vi "Actor Core.vi"(8 "error in":errorcluster, 11 "Activation in":refnum<class "Activation.lvclass">) -> (0 "error out":errorcluster, 3 "Actor out":refnum<class "Actor.lvclass">)   [LabVIEW 2018, in "Activation Actor.lvlib" / "Activation.lvclass"]
doc: "(<B>Filename</B>: Actor Framework.lvlib:Actor.lvclass:Actor Core.vi)\n\nReceives messages to the actor, reacts to them, and initiates any error handling that may shut the actor down.\n\nDescendant classes may override this VI to append parallel tasks for the actor to complete while it handles messages. Overrides use the Call Parent Method node."
uses:
  Activation.lvclass
  C:/Users/Administrator/Desktop/LabVIEW EMS/EMS Generic Actor/EMS Generic/EMS Generic.lvclass
  C:/Users/Administrator/Desktop/LabVIEW EMS/Device Communication and Control Abstract Actor/Device Communication and Control Abstract/Device Communication and Control Abstract.lvclass
  C:/Users/Administrator/Desktop/LabVIEW EMS/Optimization/Startup Optimization Actor/Startup Optimization/Startup Optimization.lvclass
  C:/Users/Administrator/Desktop/LabVIEW EMS/Optimization/Generic Optimization Actor/Generic Optimization/Generic Optimization.lvclass
  C:/Program Files (x86)/National Instruments/LabVIEW 2018/vi.lib/ActorFramework/Actor/Actor.lvclass
  <vilib>/ActorFramework/Actor/Actor.lvclass
  Controls/Activation State.ctl
  <vilib>/ORNL/CSEISMIC DDS/CSEISMIC DDS Base/Data Types/Controls/DeviceID.ctl
  EMS Generic Actor/EMS Generic/EMS Generic.lvclass/EMS Generic.ctl
  EMS Generic Actor/EMS Generic/Controls/Device Information Cluster.ctl
  EMS Generic Actor/EMS Generic/Controls/Device State.ctl
  <vilib>/ORNL/CSEISMIC DDS/CSEISMIC DDS Base/Data Types/DER_VF.ctl
  Startup Optimization Actor/Startup Optimization/Startup Optimization.lvclass/Startup Optimization.ctl
  <vilib>/ActorFramework/Actor/Actor.lvclass/Actor.ctl
  Device Communication and Control Abstract Actor/Device Communication and Control Abstract/Device Communication and Control Abstract.lvclass/Device Communication and Control Abstract.ctl
  Device Communication and Control Abstract Actor/Device Communication and Control Abstract Messages/Set DER VF Msg/Set DER VF Msg.lvclass/Set DER VF Msg.ctl
  <vilib>/ActorFramework/Message Enqueuer/Message Enqueuer.lvclass/Message Enqueuer.ctl
  <vilib>/ORNL/CSEISMIC DDS/CSEISMIC DDS Base/Data Types/Relay_Control.ctl
  Device Communication and Control Abstract Actor/Device Communication and Control Abstract Messages/Set Relay Control Msg/Set Relay Control Msg.lvclass/Set Relay Control Msg.ctl
  <vilib>/ORNL/CSEISMIC DDS/CSEISMIC DDS Base/Data Types/Load_Control.ctl
  Device Communication and Control Abstract Actor/Device Communication and Control Abstract Messages/Set Load Control Msg/Set Load Control Msg.lvclass/Set Load Control Msg.ctl
  Device Communication and Control Abstract Actor/Device Communication and Control Abstract Messages/Set DER VF Msg/Send Set DER VF.vi
  <vilib>/ActorFramework/Actor/Read Caller Enqueuer.vi
  Device Communication and Control Abstract Actor/Device Communication and Control Abstract Messages/Set PCC Transition Msg/Send Set PCC Transition.vi
  Device Communication and Control Abstract Actor/Device Communication and Control Abstract Messages/Set Relay Control Msg/Send Set Relay Control.vi
  Device Communication and Control Abstract Actor/Device Communication and Control Abstract Messages/Set Load Control Msg/Send Set Load Control.vi
  <vilib>/ActorFramework/Message Enqueuer/Init from Existing Queue.vi
  <vilib>/ActorFramework/Message Enqueuer/Enqueue.vi
  Device Communication and Control Abstract Actor/Device Communication and Control Abstract/Device Communication and Control Abstract.lvclass
  Device Communication and Control Abstract Actor/Device Communication and Control Abstract Messages/Set DER VF Msg/Set DER VF Msg.lvclass
  C:/Program Files (x86)/National Instruments/LabVIEW 2018/vi.lib/ActorFramework/Message/Message.lvclass
  Device Communication and Control Abstract Actor/Device Communication and Control Abstract Messages/Set Relay Control Msg/Set Relay Control Msg.lvclass
  Device Communication and Control Abstract Actor/Device Communication and Control Abstract Messages/Set Load Control Msg/Set Load Control Msg.lvclass
  <vilib>/ActorFramework/Stop Msg/Stop Msg.lvclass
  <vilib>/ActorFramework/Message Priority Queue/Priority Enqueue.vi
  Startup Optimization Actor/Startup Optimization/Startup Optimization.lvclass
  <vilib>/ORNL/CSEISMIC DDS/CSEISMIC DDS Base/Data Types/PCC_Transition.ctl
  <vilib>/ActorFramework/Message Enqueuer/Message Enqueuer.lvclass
  <vilib>/ORNL/CSEISMIC DDS/CSEISMIC DDS Base/CSEISMIC DDS.lvclass
  Utilities/Status Messaging.llb/Status Messaging.lvlib
  EMS Generic Actor/EMS Generic/EMS Generic.lvclass
  Generic Optimization Actor/Generic Optimization/Generic Optimization.lvclass
panel:
  out "Status":T1
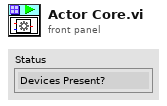
[diagram p1: front panel]
types:
  T1 = typedef "Activation Actor.lvlib/Activation.lvclass/Activation State.ctl" = enum16{"Devices Present?", "Group Devices", "Set VF Device", "Resync", "Close Relays", "Activate Loads", "Activate DERs", "Success", "Failure"}
  T2 = typedef "CSEISMIC DDS.lvlib/CSEISMIC DDS.lvclass/DeviceID.ctl" = string
  T3 = enum32{"Invalid", "Standard", "Closed", "Hidden", "Minimized", "Maximized"}
  T4 = typedef "EMS Generic Actor.lvlib/EMS Generic.lvclass/Device Information Cluster.ctl" = cluster{"Device State":T5, "data":variant}
  T5 = typedef "EMS Generic Actor.lvlib/EMS Generic.lvclass/Device State.ctl" = enum16{"Invalid", "Clear", "DevIDs in Config", "DevIDs on uGrid", "DevIDs not on uGrid", "Update IED_Status", "Update DER_Status", "Update DER_Measurement", "Update SmartRelay_Measurement"}
  T6 = typedef "CSEISMIC DDS.lvlib/CSEISMIC DDS.lvclass/DER_VF.ctl" = cluster{"DeviceID":T2}
  T7 = typedef "EMS Generic Actor.lvlib/EMS Generic.lvclass/Global Configuration.ctl" = cluster{"Microgrid ID":u8, "VF Device ID":T2, "Ongrid VF Priority":T2[], "Offgrid VF Priority":T2[], "AutoSwap Offgrid VF":u32, "AutoSwap Offgrid VF Delay (sec)":dbl, "AutoSwap Resynch VF":u32, "PCC Device ID":T2, "Device ID Array":T2[], "Nominal Voltage":dbl, "Nominal Frequency":dbl, "Resynch Timeout (sec)":dbl, "Island VF Activate Timeout (sec)":dbl, "Island PCC Target Power (kW)":dbl, "Island PCC Target Power Timeout (sec)":dbl, "Island Grid Settle Time (sec)":dbl, "Island PCC Failure Timeout (sec)":dbl, "Activation Devices Present Timeout (sec)":dbl, "Activation Devices Activated Timeout (sec)":dbl, "Blackstart VF GenMode Wait (sec)":dbl, "Blackstart VF DERCtrl Wait (sec)":dbl, "Blackstart Success Wait (sec)":dbl, "OnGrid Optimization Delay (sec)":dbl, "OffGrid Optimization Delay (sec)":dbl, "Resynch Frequency (Hz)":dbl, "Optimization Path":string}
  T8 = typedef "CSEISMIC DDS.lvlib/CSEISMIC DDS.lvclass/PCC_Transition.ctl" = cluster{"DeviceID":T2, "Island":bool, "Resynchronize":bool}
  T9 = typedef "CSEISMIC DDS.lvlib/CSEISMIC DDS.lvclass/IED_Status.ctl" = cluster{"DeviceID":T2, "Timestamp":T10, "MicrogridID":u8, "Active":bool, "Inactive":bool, "Error":i32, "Fault":bool, "ErrorString":string}
  T10 = typedef "CSEISMIC DDS.lvlib/CSEISMIC DDS.lvclass/Timestamp.ctl" = cluster{"Seconds":u64, "Remainder":u64}
  T11 = typedef "CSEISMIC DDS.lvlib/CSEISMIC DDS.lvclass/Relay_Control.ctl" = cluster{"DeviceID":T2, "Activate":bool, "Deactivate":bool}
  T12 = typedef "CSEISMIC DDS.lvlib/CSEISMIC DDS.lvclass/Load_Control.ctl" = cluster{"DeviceID":T2, "Activate":bool, "Deactivate":bool}
  T13 = typedef "CSEISMIC DDS.lvlib/CSEISMIC DDS.lvclass/SmartRelay_Measurement.ctl" = cluster{"DeviceID":T2, "PrimaryVoltage":dbl[], "SecondaryVoltage":dbl[], "Current":dbl[], "RealPower":dbl[], "ReactivePower":dbl[], "LineConfig":u8[], "Frequency":dbl}
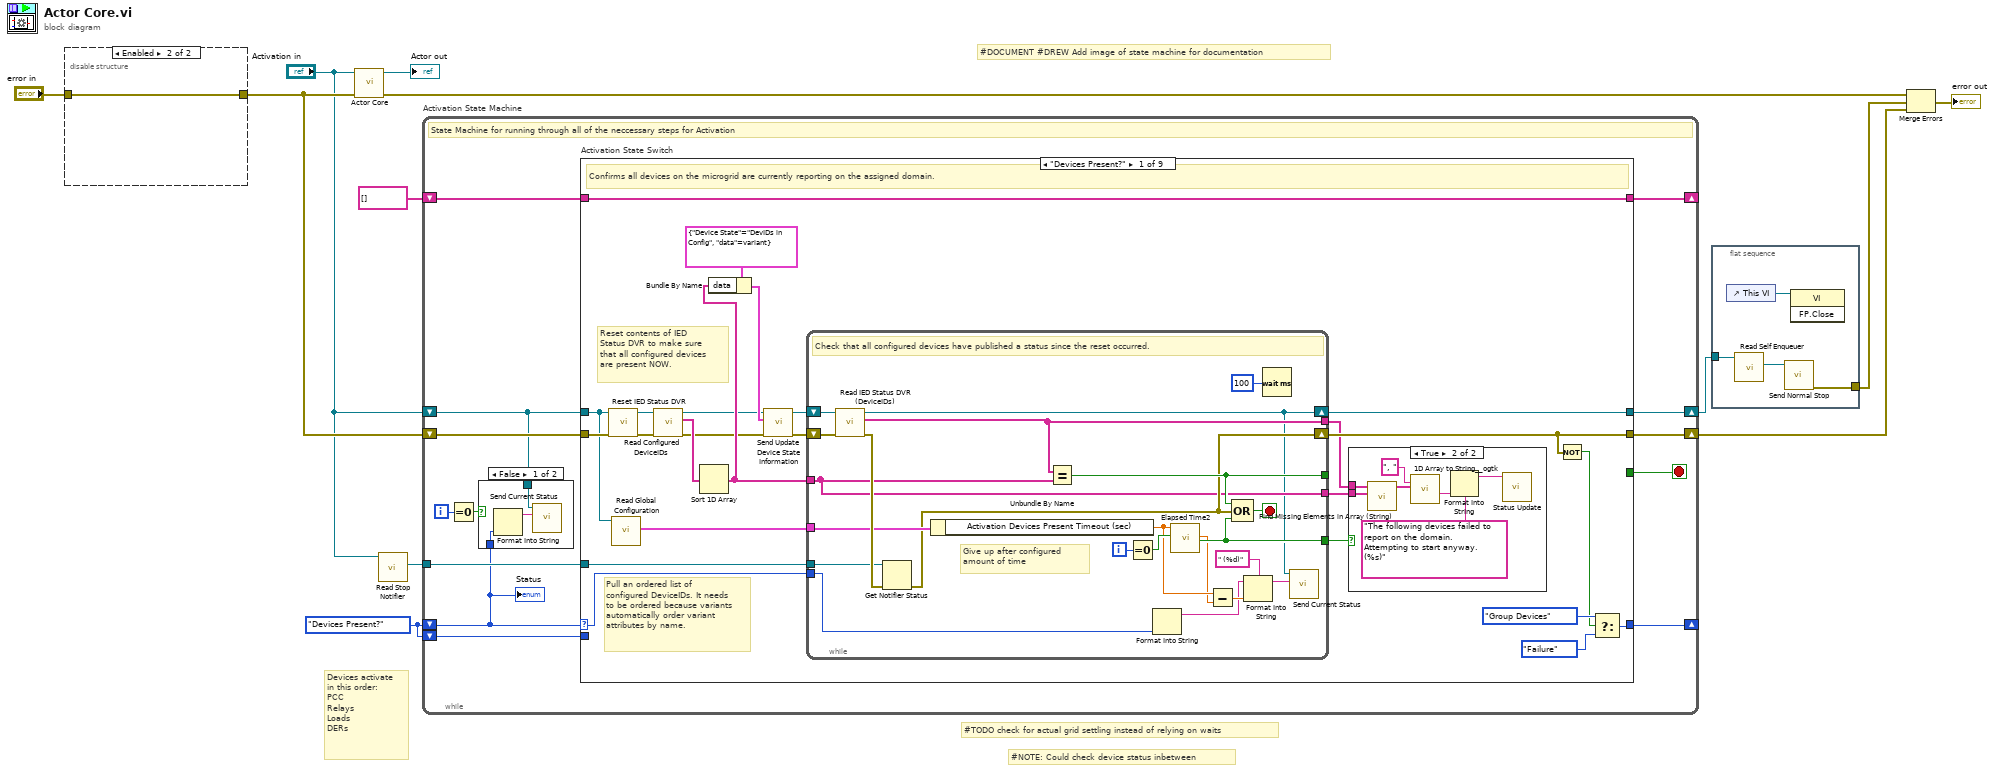
[diagram p0: block diagram]
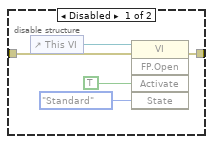
[diagram p2: hidden frame]
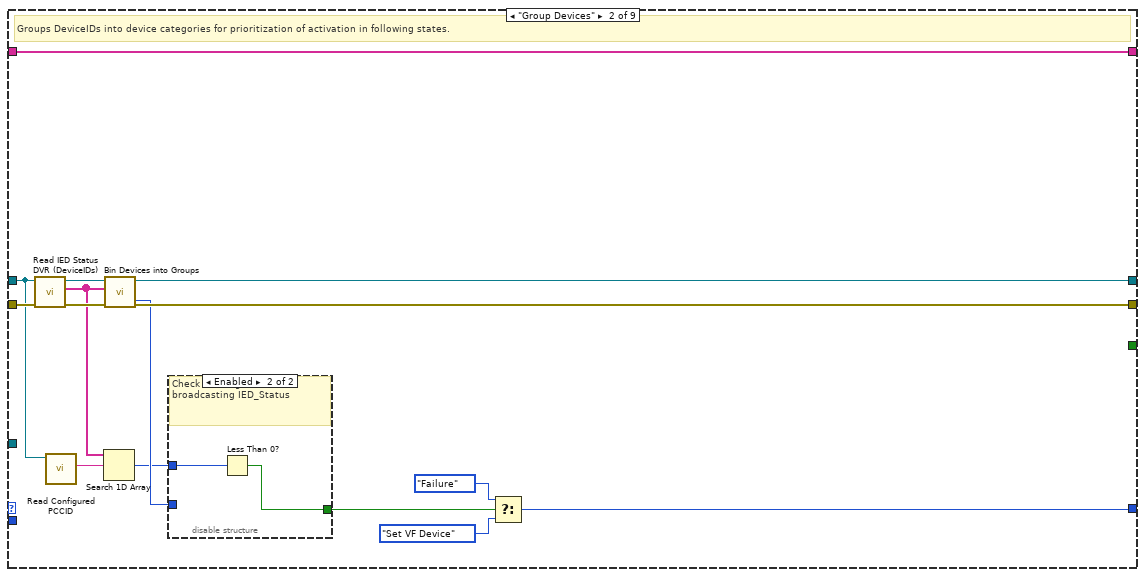
[diagram p5: hidden frame]
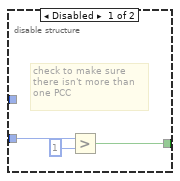
[diagram p6: hidden frame]
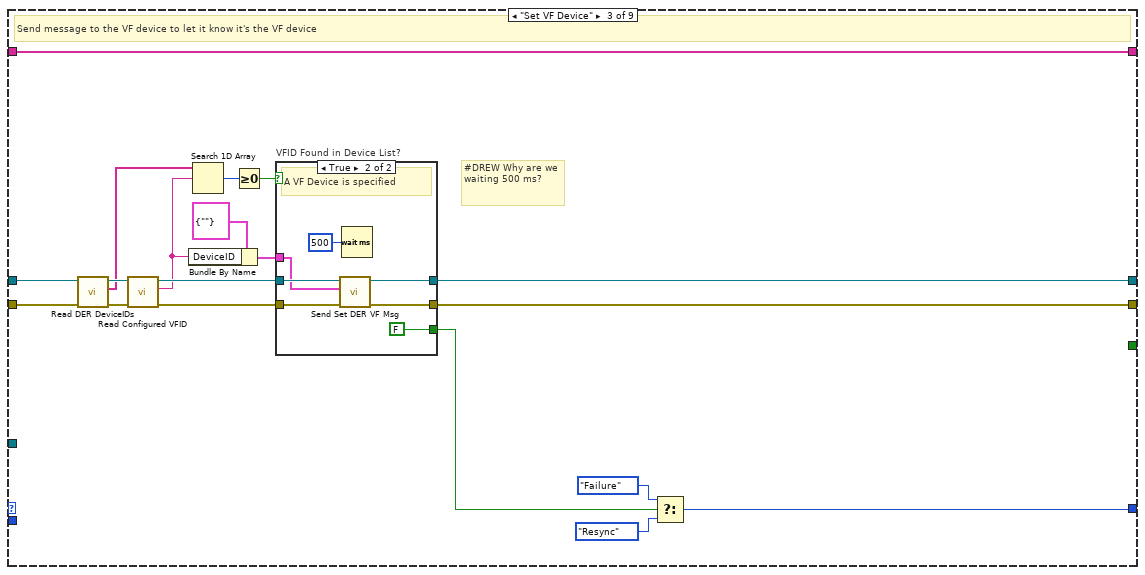
[diagram p7: hidden frame]
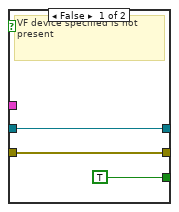
[diagram p8: hidden frame]
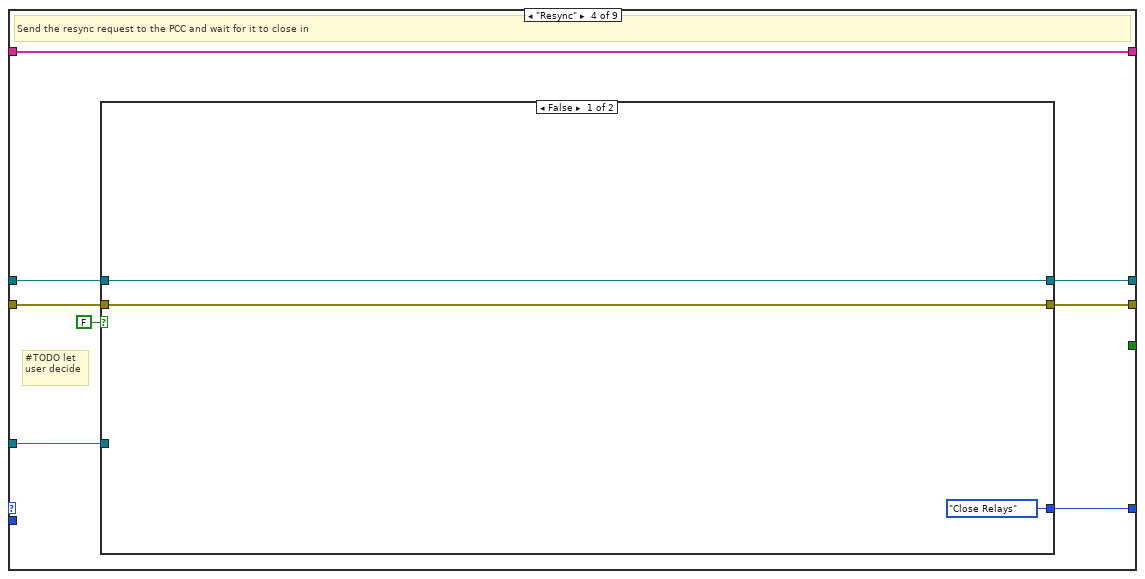
[diagram p9: hidden frame]
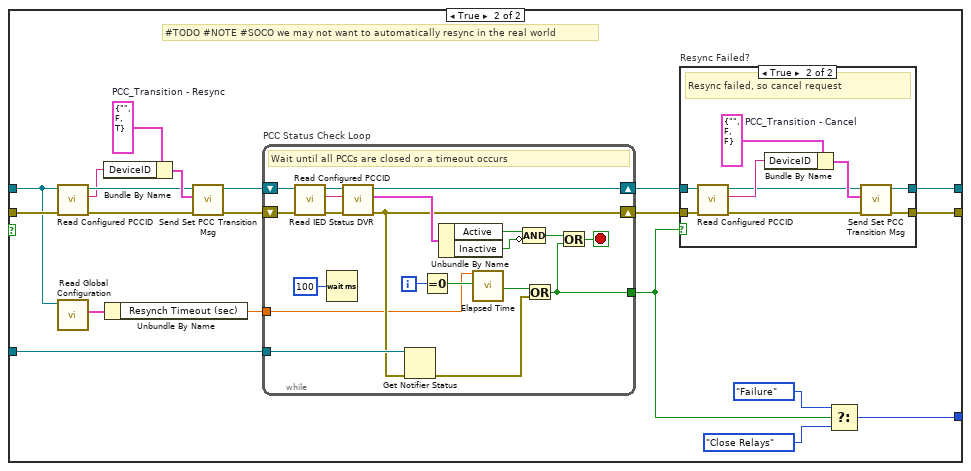
[diagram p10: hidden frame]
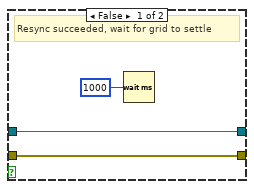
[diagram p11: hidden frame]
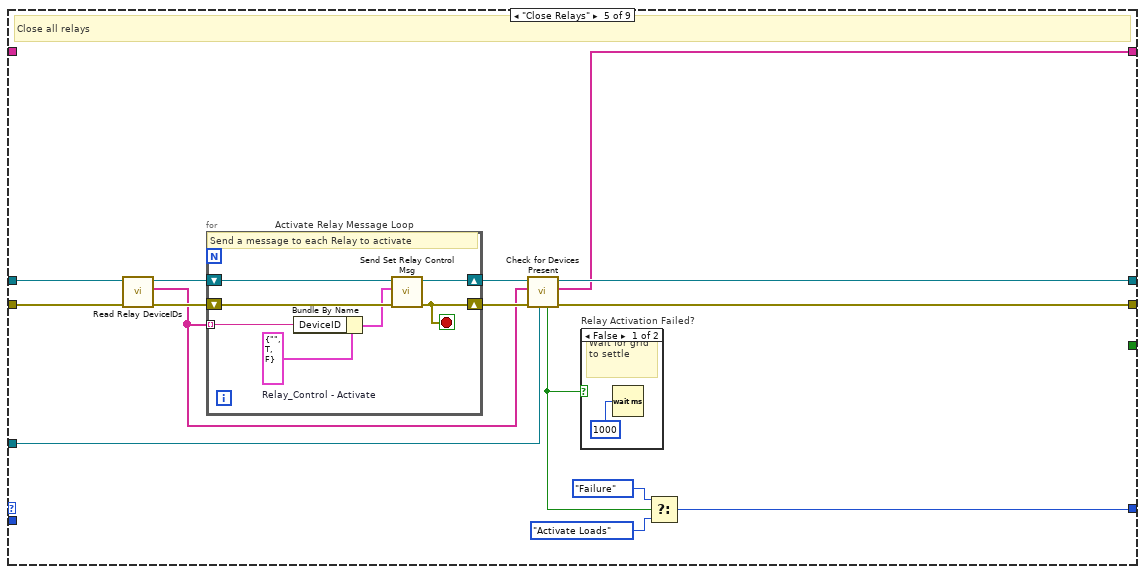
[diagram p12: hidden frame]
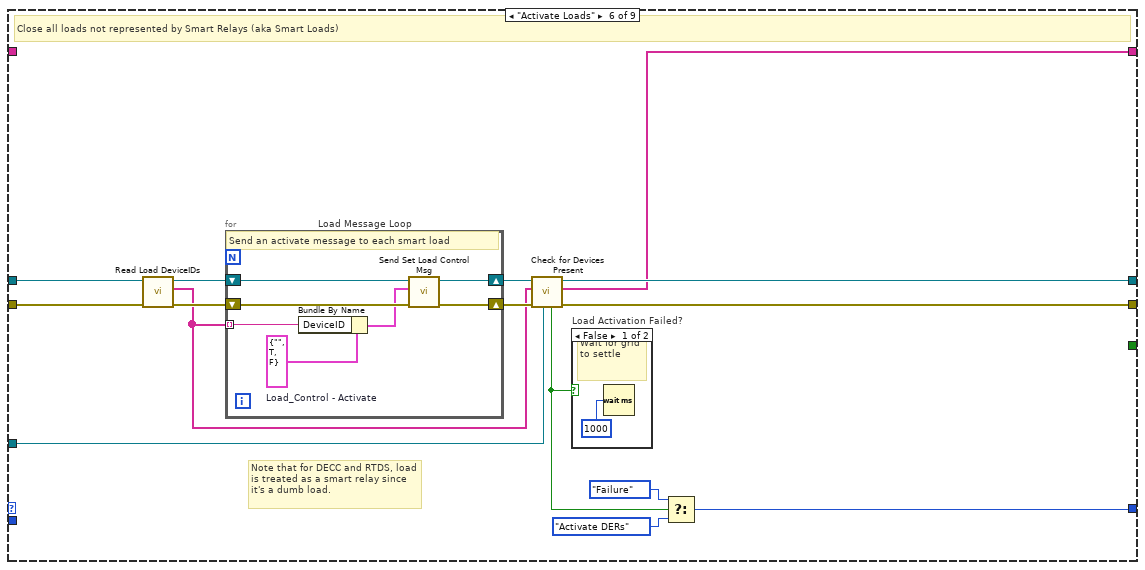
[diagram p14: hidden frame]
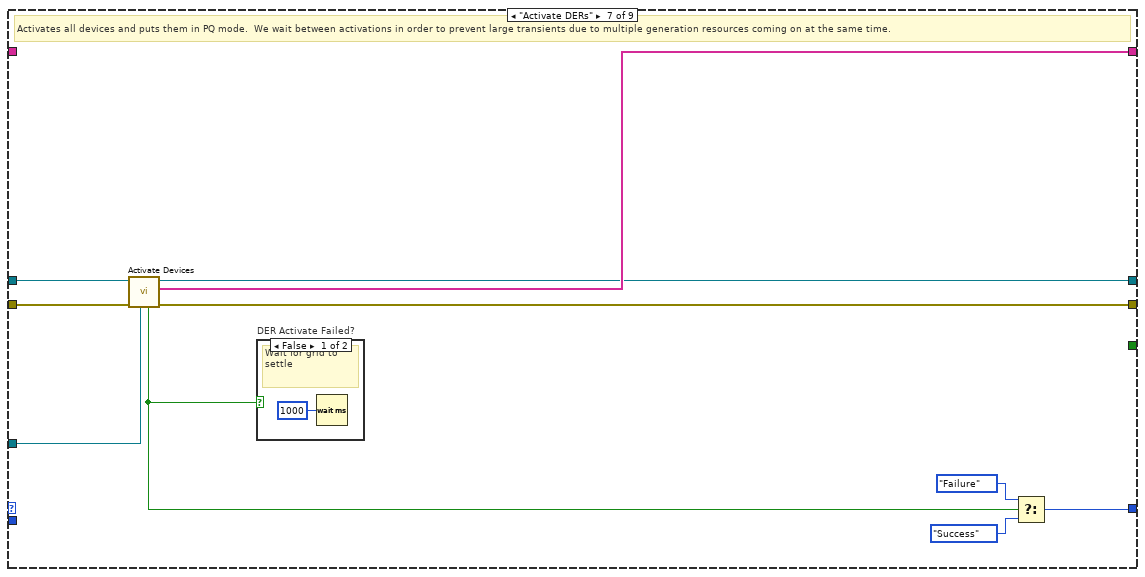
[diagram p16: hidden frame]
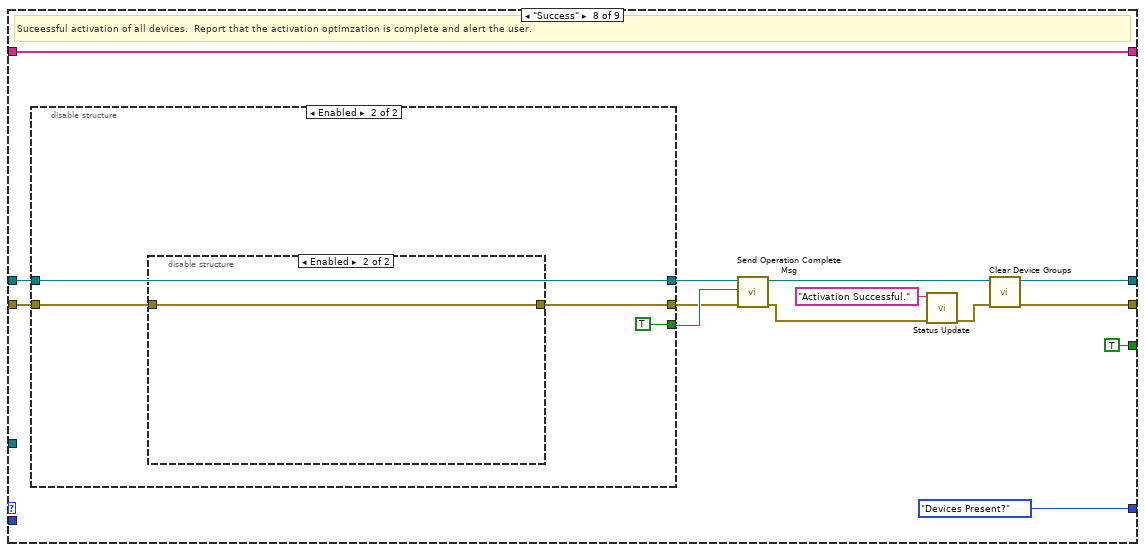
[diagram p18: hidden frame]
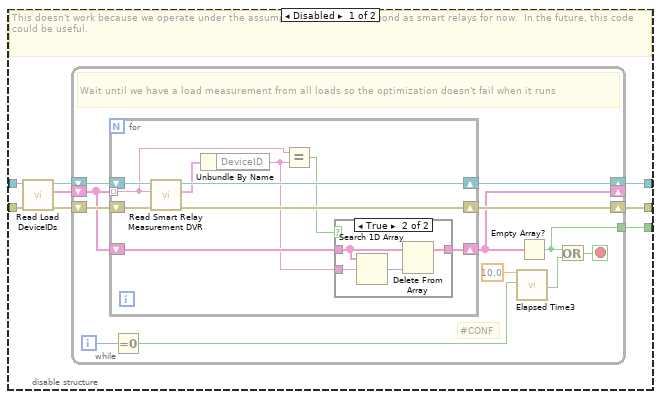
[diagram p19: hidden frame]
diagram:
  w11 = Activation_State."Devices Present?"
  # "#DOCUMENT #DREW Add image of state machine for documentation"
  # "#NOTE: Could check device status inbetween"
  # "#TODO check for actual grid settling instead of relying on waits"
  # "Devices activate in this order:\nPCC\nRelays\nLoads\nDERs"
  n1 = disable-structure shown="Enabled" {
    disable-tunnel: "error in" -> [w14 w18]
    disable-tunnel: [w13 w18] -> w3
    frame Disabled {
      n2 = control-ref of="This VI"() -> (w17:refnum<vi>)
      n3 = invoke class="VI" method="FP.Open"(reference=w17, error in=w14, "Activate"=TRUE ("Activate?"), "State"=T3."Standard") -> (error out=w13:errorcluster)  [unwired: 1 in, 4 out]
    }
    frame Enabled {
    }
  }
  n4 = call-parent "Actor Core.vi"("error in"=w3, "Actor in"="Activation in") -> ("error out"=w12:errorcluster, "Actor out"=→"Actor out":refnum<class "Actor.lvclass">)  [unwired: 8 in]
  n5 = call "Read Stop Notifier.vi"("EMS Generic in"="Activation in") -> ("stop"=w4:refnum<notifier>)  [unwired: 9 in, 1 out]
  n6 = while "Activation State Machine" {
    shift-right: [w31] -> _
    shift-left: w11 -> [w21]
    shift-left: w11 -> [w29]
    tunnel: w4 -> [w28]
    shift-right: [w27] -> _
    shift-left: T2[] [] -> [w26]
    shift-right: [w25] -> w6
    shift-left: w3 -> [w24]
    shift-right: [w23] -> w7
    shift-left: "Activation in" -> [w22]
    i -> [w20]
    stop <- w30 stop-if-true
    # "State Machine for running through all of the neccessary steps for Activation"
    n7 = Equal To 0?(x=w20) -> (x = 0?=w19:bool)
    n8 = case shown="False" w19 {
      tunnel: w22 -> [w34 _]
      tunnel: w21 -> [w33 _]
      frame False {
        n9 = Format Into String(w33) -> (resulting string=w32:string)  [unwired: 3 in, 1 out]
        n10 = call "Send Current Status.vi"("Current Status"=w32, "Device Communication and Control Abstract in"=w34) -> ()  [unwired: 8 in, 2 out]
      }
      frame True {
      }
    }
    n11 = case "Activation State Switch" shown="\"Devices Present?\"" w21 {
      selector: w21 -> [w38 _ _ _ _ _ _ _ _]
      tunnel: [w57 w103 w123 w145 w213 w236 w256 Activation_State."Devices Present?" Activation_State."Devices Present?"] -> w31
      tunnel: w22 -> [w50 w90 w113 w139 w205 w228 w248 w263 w325]
      tunnel: [_ _ _ _ _ _ _ TRUE TRUE] -> w30
      tunnel: w29 -> [_ _ _ _ _ _ _ _ w332]
      tunnel: w28 -> [w54 _ _ w144 w210 w232 w247 _ _]
      tunnel: [w55 w99 w121 w143 w208 w230 w252 w268 w328] -> w27
      tunnel: w26 -> [w55 w99 w121 w143 _ _ _ w268 w328]
      tunnel: [w48 w94 w115 w141 w207 w233 w253 w264 w318] -> w25
      tunnel: w24 -> [w52 w98 w112 w140 w203 w226 w249 w262 w320]
      tunnel: [w44 w97 w117 w142 w212 w235 w250 w266 w321] -> w23
      frame "Devices Present?" {
        # "Pull an ordered list of configured DeviceIDs. It needs to be ordered because variants automatically order variant attributes by name."
        # "Reset contents of IED Status DVR to make sure that all configured devices are present NOW."
        # "Confirms all devices on the microgrid are currently reporting on the assigned domain."
        n12 = call "Reset IED Status DVR.vi"("error in"=w52, "SCADA in"=w50) -> ("error out"=w51:errorcluster, "dup SCADA out"=w53:refnum<class "Activation.lvclass">)  [unwired: 8 in]
        n13 = call "Read Global Configuration.vi"("EMS Generic in"=w50) -> ("Global Configuration"=w49:T7)  [unwired: 8 in, 2 out]
        n14 = call "Read Configured DeviceIDs.vi"("error in"=w51, "EMS Generic in"=w53) -> ("error out"=w36:errorcluster, "DeviceIDs"=w59:T2[], "EMS Generic out"=w39:refnum<class "Activation.lvclass">)  [unwired: 7 in]
        n15 = Sort 1D Array(array=w59) -> (sorted array=w40:T2[])
        n16 = Bundle By Name(cluster=T4 {"Device State"=enum."DevIDs in Config", "data"=variant} ("Device State Information"), "data"=w40) -> (w41:T4)
        n17 = call "Send Update Device State Information.vi"("error in (no error)"=w36, "Device State Information"=w41, "Device Communication and Control Abstract in"=w39) -> ("error out"=w35:errorcluster, "Device Communication and Control Abstract out"=w37:refnum<class "Activation.lvclass">)  [unwired: 7 in]
        n18 = while {
          tunnel: w40 -> [w75]
          shift-right: [w77] -> w48
          shift-left: w35 -> [w81]
          tunnel: [w85] -> _
          tunnel: w54 -> [w86]
          shift-right: [w67] -> w44
          shift-left: w37 -> [w80]
          tunnel: w49 -> [w79]
          tunnel: [w78] -> w46
          tunnel: [w76] -> w43
          tunnel: [w75] -> w45
          tunnel: w38 -> [w70]
          i -> [w83]
          stop <- w84 stop-if-true
          # "Give up after configured amount of time"
          # "Check that all configured devices have published a status since the reset occurred."
          n19 = call "Read IED Status DVR (DeviceIDs).vi"("error in"=w81, "EMS Generic in"=w80) -> ("error out"=w88:errorcluster, "DeviceID Array"=w76:T2[], "EMS Generic out"=w67:refnum<class "Activation.lvclass">)  [unwired: 7 in]
          n20 = Get Notifier Status(notifier=w86, error in (no error)=w88) -> (error out=w77:errorcluster)  [unwired: 4 out]
          n21 = Unbundle By Name(w79) -> ("Activation Devices Present Timeout (sec)"=w73:dbl)
          n22 = Equal?(x=w76, y=w75) -> (x = y?=w85:bool)
          n23 = Equal To 0?(x=w83) -> (x = 0?=w82:bool)
          n24 = Format Into String(w70) -> (resulting string=w69:string)  [unwired: 3 in, 1 out]
          n25 = call "Elapsed Time2"("Time Target (s)"=w73, "Reset"=w82) -> ("Elapsed Time (s)"=w72:dbl, "Time has Elapsed"=w78:bool)  [unwired: 10 in, 6 out]
          n26 = Subtract(x=w73, y=w72) -> (x-y=w71:dbl)
          n27 = Compound Arithmetic op=OR(w85, w77, w78) -> (w84:bool)
          n28 = Format Into String(format string=" (%d)", initial string=w69, w71) -> (resulting string=w74:string)  [unwired: 1 in, 1 out]
          n29 = Wait (ms)(milliseconds to wait=u32 100) -> ()  [unwired: 1 out]
          n30 = call "Send Current Status.vi"("Current Status"=w74, "Device Communication and Control Abstract in"=w67) -> ()  [unwired: 8 in, 2 out]
        }
        n31 = case shown="True" w46 {
          tunnel: w45 -> [_ w66]
          tunnel: w43 -> [_ w65]
          frame False {
          }
          frame True {
            n32 = call "Find Missing Elements in Array (String).vi"("Full Array"=w66, "Partial Array"=w65) -> ("Missing Elements"=w63:T2[])  [unwired: 9 in]
            n33 = call <userlib>:"1D Array to String__ogtk.vi"("delimiter (Tab)"=", ", "Array of Strings"=w63) -> ("delimited string"=w62:string)  [unwired: 9 in]
            n34 = Format Into String(format string="The following devices failed to report on the domain.  Attempting to start anyway. (%s)", w62) -> (resulting string=w60:string)  [unwired: 2 in, 1 out]
            n35 = call "Status Update.vi"("Status Update"=w60) -> ()  [unwired: 9 in, 2 out]
          }
        }
        n36 = Not(x=w48) -> (.not. x?=w47:bool)
        n37 = Select(t=Activation_State."Group Devices", s=w47, f=Activation_State."Failure") -> (s? t:f=w57:T1)
      }
      frame "Group Devices" {
        # "Groups DeviceIDs into device categories for prioritization of activation in following states."
        n38 = call "Read IED Status DVR (DeviceIDs).vi"("error in"=w98, "EMS Generic in"=w90) -> ("error out"=w95:errorcluster, "DeviceID Array"=w92:T2[], "EMS Generic out"=w96:refnum<class "Activation.lvclass">)  [unwired: 7 in]
        n39 = call "Read Configured PCCID.vi"("EMS Generic in"=w90) -> ("PCCID"=w91:T2)  [unwired: 8 in, 2 out]
        n40 = Search 1D Array(1D array=w92, element=w91) -> (index of element=w89:i32)  [unwired: 1 in]
        n41 = call "Bin Devices into Groups.vi"("error in (no error)"=w95, "DeviceID Array"=w92, "Startup Optimization in"=w96) -> ("error out"=w94:errorcluster, "Startup Optimization out"=w97:refnum<class "Activation.lvclass">, "Number of PCCs"=w93:i16)  [unwired: 6 in]
        n42 = disable-structure shown="Enabled" {
          disable-tunnel: [w105 w107] -> w100
          disable-tunnel: w93 -> [w104 _]
          disable-tunnel: w89 -> [_ w108]
          frame Disabled {
            # "check to make sure there isn't more than one PCC"
            n43 = Greater?(x=w104, y=i16 1) -> (0:w105:bool)
          }
          frame Enabled {
            # "Check if configured PCC is broadcasting IED_Status"
            n44 = Less Than 0?(x=w108) -> (x < 0?=w107:bool)
          }
        }
        n45 = Select(t=Activation_State."Failure", s=w100, f=Activation_State."Set VF Device") -> (s? t:f=w103:T1)
      }
      frame "Set VF Device" {
        # "#DREW Why are we waiting 500 ms?"
        # "Send message to the VF device to let it know it's the VF device"
        n46 = call "Read DER DeviceIDs.vi"("error in"=w112, "Startup Optimization in"=w113) -> ("error out"=w111:errorcluster, "DERs"=w114:T2[], "Startup Optimization out"=w126:refnum<class "Activation.lvclass">)  [unwired: 7 in]
        n47 = call "Read Configured VFID.vi"("error in"=w111, "EMS Generic in"=w126) -> ("error out"=w116:errorcluster, "VFID"=w118:T2, "EMS Generic out"=w127:refnum<class "Activation.lvclass">)  [unwired: 7 in]
        n48 = Bundle By Name(cluster=T6 {"DeviceID"=""} ("DER_VF"), "DeviceID"=w118) -> (w119:T6)
        n49 = Search 1D Array(1D array=w114, element=w118) -> (index of element=w110:i32)  [unwired: 1 in]
        n50 = Greater Or Equal To 0?(x=w110) -> (x >= 0?=w109:bool)
        n51 = case "VFID Found in Device List?" shown="True" w109 {
          tunnel: [TRUE FALSE] -> w122
          tunnel: w119 -> [_ w134]
          tunnel: w127 -> [w129 w135]
          tunnel: [w129 w133] -> w117
          tunnel: w116 -> [w128 w132]
          tunnel: [w128 w131] -> w115
          frame False {
            # "VF device specified is not present"
          }
          frame True {
            # "A VF Device is specified"
            n52 = call "Send Set DER VF Msg.vi"("error in"=w132, "DER_VF"=w134, "SCADA Sub Abstract in"=w135) -> ("error out"=w131:errorcluster, "dup SCADA Sub Abstract"=w133:refnum<class "Activation.lvclass">)  [unwired: 7 in]
            n53 = Wait (ms)(milliseconds to wait=u32 500) -> ()  [unwired: 1 out]
          }
        }
        n54 = Select(t=Activation_State."Failure", s=w122, f=Activation_State."Resync") -> (s? t:f=w123:T1)
      }
      frame "Resync" {
        # "#TODO let user decide"
        # "Send the resync request to the PCC and wait for it to close in"
        n55 = case shown="False" FALSE {
          tunnel: [Activation_State."Close Relays" w167] -> w145
          tunnel: w144 -> [_ w164]
          tunnel: [w147 w161] -> w142
          tunnel: [w146 w160] -> w141
          tunnel: w140 -> [w146 w153]
          tunnel: w139 -> [w147 w151]
          frame False {
          }
          frame True {
            w165 = T8 {"DeviceID"="", "Island"=FALSE, "Resynchronize"=TRUE}  # PCC_Transition - Resync
            # "#TODO #NOTE #SOCO we may not want to automatically resync in the real world"
            n56 = call "Read Configured PCCID.vi"("error in"=w153, "EMS Generic in"=w151) -> ("error out"=w152:errorcluster, "PCCID"=w149:T2, "EMS Generic out"=w150:refnum<class "Activation.lvclass">)  [unwired: 7 in]
            n57 = call "Read Global Configuration.vi"("EMS Generic in"=w151) -> ("Global Configuration"=w155:T7)  [unwired: 8 in, 2 out]
            n58 = Bundle By Name(cluster=w165, "DeviceID"=w149) -> (w156:T8)
            n59 = Unbundle By Name(w155) -> ("Resynch Timeout (sec)"=w154:dbl)
            n60 = call "Send Set PCC Transition Msg.vi"("error in"=w152, "PCC_Transition"=w156, "SCADA Sub Abstract in"=w150) -> ("error out"=w158:errorcluster, "dup SCADA Sub Abstract"=w157:refnum<class "Activation.lvclass">)  [unwired: 7 in]
            n61 = while "PCC Status Check Loop" {
              tunnel: [w199] -> w159
              tunnel: w164 -> [w198]
              shift-right: [w190] -> w163
              shift-left: w158 -> [w188]
              shift-right: [w191] -> w162
              shift-left: w157 -> [w187]
              tunnel: w154 -> [w189]
              i -> [w197]
              stop <- w200 stop-if-true
              # "Wait until all PCCs are closed or a timeout occurs"
              n62 = call "Read Configured PCCID.vi"("error in"=w188, "EMS Generic in"=w187) -> ("error out"=w184:errorcluster, "PCCID"=w185:T2, "EMS Generic out"=w186:refnum<class "Activation.lvclass">)  [unwired: 7 in]
              n63 = Wait (ms)(milliseconds to wait=u32 100) -> ()  [unwired: 1 out]
              n64 = call "Read IED Status DVR.vi"("error in"=w184, "DeviceID"=w185, "EMS Generic in"=w186) -> ("error out"=w190:errorcluster, "IED_Status"=w194:T9, "EMS Generic out"=w191:refnum<class "Activation.lvclass">)  [unwired: 5 in, 1 out]
              n65 = Get Notifier Status(notifier=w198, error in (no error)=w190) -> (error out=w192:errorcluster)  [unwired: 4 out]
              n66 = Equal To 0?(x=w197) -> (x = 0?=w196:bool)
              n67 = Unbundle By Name(w194) -> ("Active"=w183:bool, "Inactive"=w182:bool)
              n68 = call "Elapsed Time"("Time Target (s)"=w189, "Reset"=w196) -> ("Time has Elapsed"=w193:bool)  [unwired: 10 in, 7 out]
              n69 = Compound Arithmetic op=AND(w183, invert w182) -> (w181:bool)
              n70 = Or(x=w193, y=w192) -> (x .or. y?=w199:bool)
              n71 = Or(x=w181, y=w199) -> (x .or. y?=w200:bool)
            }
            n72 = case "Resync Failed?" shown="True" w159 {
              tunnel: w162 -> [w171 w176]
              tunnel: [w171 w178] -> w161
              tunnel: w163 -> [w170 w175]
              tunnel: [w170 w179] -> w160
              frame False {
                # "Resync succeeded, wait for grid to settle"
                n73 = Wait (ms)(milliseconds to wait=u32 1000) -> ()  [unwired: 1 out]
              }
              frame True {
                w180 = T8 {"DeviceID"="", "Island"=FALSE, "Resynchronize"=FALSE}  # PCC_Transition - Cancel
                # "Resync failed, so cancel request"
                n74 = call "Read Configured PCCID.vi"("error in"=w175, "EMS Generic in"=w176) -> ("error out"=w174:errorcluster, "PCCID"=w173:T2, "EMS Generic out"=w172:refnum<class "Activation.lvclass">)  [unwired: 7 in]
                n75 = Bundle By Name(cluster=w180, "DeviceID"=w173) -> (w177:T8)
                n76 = call "Send Set PCC Transition Msg.vi"("error in"=w174, "PCC_Transition"=w177, "SCADA Sub Abstract in"=w172) -> ("error out"=w179:errorcluster, "dup SCADA Sub Abstract"=w178:refnum<class "Activation.lvclass">)  [unwired: 7 in]
              }
            }
            n77 = Select(t=Activation_State."Failure", s=w159, f=Activation_State."Close Relays") -> (s? t:f=w167:T1)
          }
        }
      }
      frame "Close Relays" {
        # "Close all relays"
        n78 = call "Read Relay DeviceIDs.vi"("error in (no error)"=w203, "Startup Optimization in"=w205) -> ("error out"=w202:errorcluster, "Relays"=w201:T2[], "Startup Optimization out"=w204:refnum<class "Activation.lvclass">)  [unwired: 7 in]
        n79 = for "Activate Relay Message Loop" {
          tunnel: w201 -> [w222] mode=indexing
          shift-right: [w219] -> w211
          shift-left: w202 -> [w218]
          shift-right: [w220] -> w206
          shift-left: w204 -> [w221]
          stop <- w219 stop-if-true
          w223 = T11 {"DeviceID"="", "Activate"=TRUE, "Deactivate"=FALSE}  # Relay_Control - Activate
          # "Send a message to each Relay to activate"
          n80 = Bundle By Name(cluster=w223, "DeviceID"=w222) -> (w217:T11)
          n81 = call "Send Set Relay Control Msg.vi"("error in"=w218, "Relay_Control"=w217, "SCADA Sub Abstract in"=w221) -> ("error out"=w219:errorcluster, "dup SCADA Sub Abstract"=w220:refnum<class "Activation.lvclass">)  [unwired: 7 in]
        }
        n82 = call "Check for Devices Present.vi"("stop notifier reference"=w210, "error in"=w211, "Devices in"=w201, "Startup Optimization in"=w206) -> ("error out"=w207:errorcluster, "Failed Devices"=w208:T2[], "Startup Optimization out"=w212:refnum<class "Activation.lvclass">, "Time has Elapsed"=w209:bool)  [unwired: 4 in]
        n83 = case "Relay Activation Failed?" shown="False" w209 {
          frame False {
            # "Wait for grid to settle"
            n84 = Wait (ms)(milliseconds to wait=u32 1000) -> ()  [unwired: 1 out]
          }
          frame True {
          }
        }
        n85 = Select(t=Activation_State."Failure", s=w209, f=Activation_State."Activate Loads") -> (s? t:f=w213:T1)
      }
      frame "Activate Loads" {
        # "Note that for DECC and RTDS, load is treated as a smart relay since it's a dumb load."
        # "Close all loads not represented by Smart Relays (aka Smart Loads)"
        n86 = call "Read Load DeviceIDs.vi"("error in (no error)"=w226, "Startup Optimization in"=w228) -> ("error out"=w225:errorcluster, "Loads"=w224:T2[], "Startup Optimization out"=w227:refnum<class "Activation.lvclass">)  [unwired: 7 in]
        n87 = for "Load Message Loop" {
          tunnel: w224 -> [w246] mode=indexing
          shift-right: [w242] -> w234
          shift-left: w225 -> [w241]
          shift-right: [w243] -> w229
          shift-left: w227 -> [w244]
          w245 = T12 {"DeviceID"="", "Activate"=TRUE, "Deactivate"=FALSE}  # Load_Control - Activate
          # "Send an activate message to each smart load"
          n88 = Bundle By Name(cluster=w245, "DeviceID"=w246) -> (w240:T12)
          n89 = call "Send Set Load Control Msg.vi"("error in"=w241, "Load_Control"=w240, "SCADA Sub Abstract in"=w244) -> ("error out"=w242:errorcluster, "dup SCADA Sub Abstract"=w243:refnum<class "Activation.lvclass">)  [unwired: 7 in]
        }
        n90 = call "Check for Devices Present.vi"("stop notifier reference"=w232, "error in"=w234, "Devices in"=w224, "Startup Optimization in"=w229) -> ("error out"=w233:errorcluster, "Failed Devices"=w230:T2[], "Startup Optimization out"=w235:refnum<class "Activation.lvclass">, "Time has Elapsed"=w231:bool)  [unwired: 4 in]
        n91 = case "Load Activation Failed?" shown="False" w231 {
          frame False {
            # "Wait for grid to settle"
            n92 = Wait (ms)(milliseconds to wait=u32 1000) -> ()  [unwired: 1 out]
          }
          frame True {
          }
        }
        n93 = Select(t=Activation_State."Failure", s=w231, f=Activation_State."Activate DERs") -> (s? t:f=w236:T1)
      }
      frame "Activate DERs" {
        # "Activates all devices and puts them in PQ mode.  We wait between activations in order to prevent large transients due to multiple generation resources coming on at the same time."
        n94 = call "Activate Devices.vi"("stop"=w247, "error in"=w249, "Activation in"=w248) -> ("error out"=w253:errorcluster, "Failed Devices"=w252:T2[], "Activation out"=w250:refnum<class "Activation.lvclass">, "Activation Failed?"=w251:bool)  [unwired: 5 in]
        n95 = case "DER Activate Failed?" shown="False" w251 {
          frame False {
            # "Wait for grid to settle"
            n96 = Wait (ms)(milliseconds to wait=u32 1000) -> ()  [unwired: 1 out]
          }
          frame True {
          }
        }
        n97 = Select(t=Activation_State."Failure", s=w251, f=Activation_State."Success") -> (s? t:f=w256:T1)
      }
      frame "Success" {
        # "Suceessful activation of all devices.  Report that the activation optimzation is complete and alert the user."
        n98 = disable-structure shown="Enabled" {
          disable-tunnel: [w279 w309] -> w259
          disable-tunnel: w263 -> [w278 w307]
          disable-tunnel: w262 -> [w277 w310]
          disable-tunnel: [w273 w307] -> w261
          disable-tunnel: [w272 TRUE ("Operation Complete")] -> w260
          frame Disabled {
            # "This doesn't work because we operate under the assumption that Loads respond as smart relays for now.  In the future, this code could be useful."
            n99 = call "Read Load DeviceIDs.vi"("error in (no error)"=w277, "Startup Optimization in"=w278) -> ("error out"=w276:errorcluster, "Loads"=w274:T2[], "Startup Optimization out"=w275:refnum<class "Activation.lvclass">)  [unwired: 7 in]
            n100 = while {
              shift-right: [w288] -> w279
              shift-left: w276 -> [w290]
              shift-right: [w289] -> w273
              shift-left: w275 -> [w291]
              shift-right: [w283] -> _
              shift-left: w274 -> [w287]
              tunnel: [w280] -> w272
              i -> [w286]
              stop <- w281 stop-if-true
              # "#CONF"
              # "Wait until we have a load measurement from all loads so the optimization doesn't fail when it runs"
              n101 = for {
                shift-right: [w299] -> w289
                shift-left: w291 -> [w301]
                shift-right: [w298] -> w288
                shift-left: w290 -> [w300]
                tunnel: w287 -> [w296] mode=indexing
                shift-right: [w293] -> w283
                shift-left: w287 -> [w294]
                n102 = call "Read Smart Relay Measurement DVR.vi"("error in"=w300, "DeviceID"=w296, "EMS Generic in"=w301) -> ("error out"=w298:errorcluster, "SmartRelay_Measurement"=w297:T13, "EMS Generic out"=w299:refnum<class "Activation.lvclass">)  [unwired: 5 in, 1 out]
                n103 = Unbundle By Name(w297) -> ("DeviceID"=w292:T2)
                n104 = Equal?(x=w296, y=w292) -> (x = y?=w295:bool)
                n105 = case shown="True" w295 {
                  tunnel: w294 -> [w302 w304]
                  tunnel: [w302 w306] -> w293
                  tunnel: w292 -> [_ w303]
                  frame False {
                  }
                  frame True {
                    n106 = Search 1D Array(1D array=w304, element=w303) -> (index of element=w305:i32)  [unwired: 1 in]
                    n107 = Delete From Array(array=w304, index=w305) -> (array with subset deleted=w306:T2[])  [unwired: 1 in, 1 out]
                  }
                }
              }
              n108 = Equal To 0?(x=w286) -> (x = 0?=w285:bool)
              n109 = call "Elapsed Time3"("Time Target (s)"=10.0, "Reset"=w285) -> ("Time has Elapsed"=w282:bool)  [unwired: 10 in, 7 out]
              n110 = Empty Array?(array=w283) -> (empty?=w280:bool)
              n111 = Or(x=w280, y=w282) -> (x .or. y?=w281:bool)
            }
          }
          frame Enabled {
            n112 = disable-structure shown="Enabled" {
              disable-tunnel: w310 -> [w312 w314]
              disable-tunnel: [w311 w314] -> w309
              frame Disabled {
                # "#DREW this is now done in Generic Optimization.lvclass:Ensure Load Measurements Exists.vi"
                # "#DREW added 7 second wait to allow slow load reporting to actually report a value so when ongrid optimization is called, it doesn't see an empty load array.  This should be changed to wait until a load value is read (instead of having a static wait)."
                n113 = call "Error Bound Wait (ms).vi"("milliseconds to wait (100)"=u32 7000 ("milliseconds to wait"), "error in"=w312) -> ("error out"=w311:errorcluster)  [unwired: 9 in]
              }
              frame Enabled {
              }
            }
          }
        }
        n114 = call "Send Operation Complete Msg.vi"("error in"=w259, "Operation Complete"=w260, "Generic Optimization in"=w261) -> ("error out"=w258:errorcluster, "Generic Optimization out"=w267:refnum<class "Activation.lvclass">)  [unwired: 7 in]
        n115 = call "Status Update.vi"("error in"=w258, "Status Update"="Activation Successful.") -> ("error out"=w265:errorcluster)  [unwired: 8 in, 1 out]
        n116 = call "Clear Device Groups.vi"("error in"=w265, "Startup Optimization in"=w267) -> ("error out"=w264:errorcluster, "Startup Optimization out"=w266:refnum<class "Activation.lvclass">)  [unwired: 8 in]
      }
      frame "Failure", Default {
        # "Failed to activate properly.  Report that optimization failed and alert the user."
        n117 = call "Send Operation Complete Msg.vi"("error in"=w320, "Operation Complete"=FALSE ("Activation Complete"), "Generic Optimization in"=w325) -> ("error out"=w317:errorcluster, "Generic Optimization out"=w322:refnum<class "Activation.lvclass">)  [unwired: 7 in]
        n118 = Format Into String(format string="Activation Failed on %s step." ("Status Update"), w332) -> (resulting string=w331:string, error out=w327:errorcluster)  [unwired: 2 in]
        n119 = Empty Array?(array=w328) -> (empty?=w329:bool)
        n120 = case "Failed Device Array Empty?" shown="False" w329 {
          tunnel: w331 -> [w340 w345]
          tunnel: [w338 w345] -> w330
          tunnel: w328 -> [w342 _]
          tunnel: w327 -> [w337 w344]
          tunnel: [w336 w344] -> w326
          frame False {
            # "Craft failed device message"
            n121 = call <userlib>:"1D Array to String__ogtk.vi"("delimiter (Tab)"=", ", "Array of Strings"=w342) -> ("delimited string"=w339:string)  [unwired: 9 in]
            n122 = Format Into String(format string="%s (%s)", error in=w337, w340, w339) -> (resulting string=w338:string, error out=w336:errorcluster)  [unwired: 1 in]
          }
          frame True {
            # "Generic message"
          }
        }
        n123 = call "Status Update.vi"("error in"=w326, "Status Update"=w330) -> ("error out"=w323:errorcluster)  [unwired: 8 in, 1 out]
        n124 = call <vilib>:"Clear Errors.vi"("error in (no error)"=w317, "specific error code to clear (0: all)"=1) -> ("error out"=w316:errorcluster)  [unwired: 4 in, 1 out]
        n125 = call "Clear Device Groups.vi"("error in"=w323, "Startup Optimization in"=w322) -> ("error out"=w319:errorcluster, "Startup Optimization out"=w321:refnum<class "Activation.lvclass">)  [unwired: 8 in]
        n126 = Merge Errors(w316, w319) -> (w318:errorcluster)
      }
    }
    "Status" <- w21
  }
  n127 = flat-sequence {
    tunnel: w7 -> [w349]
    tunnel: [w347] -> w5
    frame #0 {
      n128 = control-ref of="This VI"() -> (w346:refnum<vi>)
      n129 = call <vilib>:"Read Self Enqueuer.vi"("Actor"=w349) -> ("Self Enqueuer"=w348:refnum<class "Message Enqueuer.lvclass">)  [unwired: 10 in]
      n130 = call <vilib>:"Send Normal Stop.vi"("Message Enqueuer"=w348) -> ("error out"=w347:errorcluster)  [unwired: 10 in]
      n131 = invoke class="VI" method="FP.Close"(reference=w346) -> ()  [unwired: 2 in, 3 out]
    }
  }
  n132 = Merge Errors(w12, w5, w6) -> (→"error out":errorcluster)
